vi "FPGA - Main.vi"() -> ()   [LabVIEW 2017]
uses:
  <vilib>/rvi/Emulation/niFpgaGetClockAttributes.vi
  <vilib>/rvi/Emulation/niFpgaSctlEmulationGetInTimedLoop.vi
  <vilib>/rvi/Emulation/niFpgaEmulationReportErrorSimple.vi
  <vilib>/rvi/eio/common/nirviEmuTemplateMethod_errors.vi
  <vilib>/rvi/interface/RandomDataEmulation/niFpgaRandomDataHandleErrors.vi
  <vilib>/rvi/Emulation/niFpgaCriticalErrorInLSC.vi
  <vilib>/eio/EIONode/EIONode.xnode
  <vilib>/rvi/DataTransferAndStorage/Container/XNode/niFpgaContainer.xnode
  <vilib>/rvi/interface/RandomDataEmulation/nirviRandomDataFpgaReadWriteTemplate.vi
panel:
  in  "Manual Log":bool
  in  "Reset":bool
  out "Loop Iteration":i32
  out "Delay":u32
  out "Data":u32[](array[numeric])
  in  "Wait(uSec)":u32
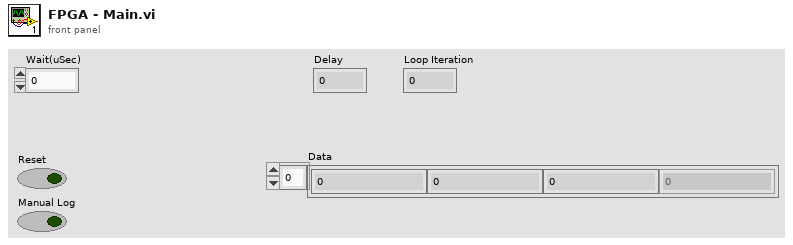
[diagram p1: front panel]
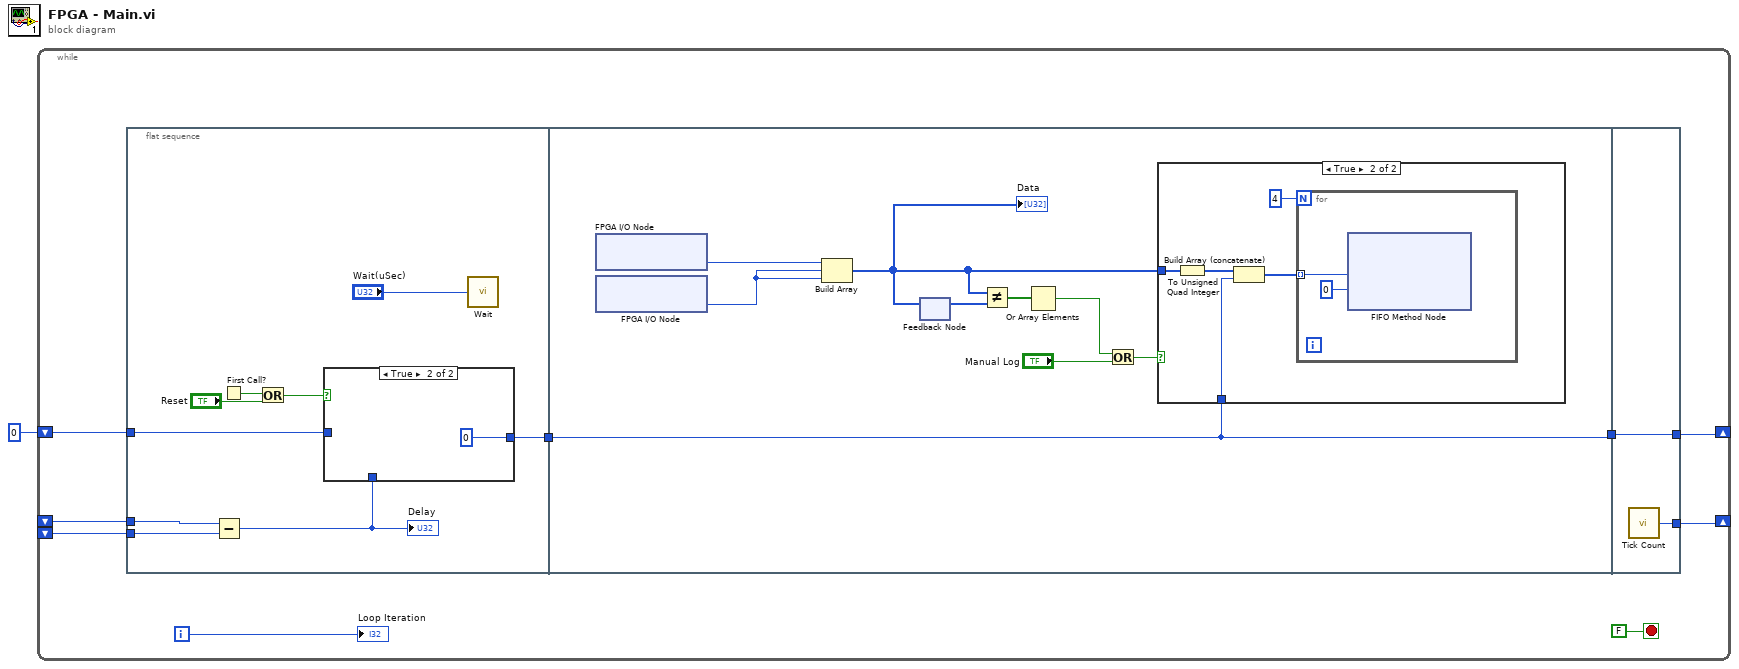
[diagram p0: block diagram]
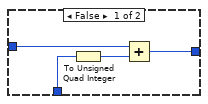
[diagram p2: hidden frame]
diagram:
  n1 = while {
    shift-right: [w9] -> _
    shift-left: _ -> [w8]
    shift-left: _ -> [w7]
    shift-right: [w2] -> _
    shift-left: u64 0 ("x-y") -> [w5]
    i -> [w6]
    stop <- FALSE stop-if-true
    n2 = flat-sequence {
      tunnel: w8 -> [w18]
      tunnel: w7 -> [w17]
      tunnel: w5 -> [w15]
      tunnel: [w14] -> w4
      tunnel: w4 -> [w29]
      tunnel: [w29] -> w3
      tunnel: [w42] -> w9
      tunnel: w3 -> [w41]
      tunnel: [w41] -> w2
      frame #0 {
        n3 = Subtract(x=w18, y=w17) -> (x-y=w16:u32)
        "Delay" <- w16
        n4 = First Call?() -> (First Call?: T/F=w13:bool)
        n5 = Or(x=w13, y="Reset") -> (x .or. y?=w11:bool)
        n6 = case shown="True" w11 {
          tunnel: w16 -> [w23 _]
          tunnel: w15 -> [w22 _]
          tunnel: [w21 u64 0] -> w14
          frame False {
            n7 = To Unsigned Quad Integer(1:w23) -> (0:w20:u64)
            n8 = Add(x=w22, y=w20) -> (x+y=w21:u64)
          }
          frame True {
          }
        }
        n9 = call "Wait"("Count(uSec)"="Wait(uSec)") -> ()  [unwired: 1 out]
      }
      frame #1 {
        n10 = xnode "FPGA I/O Node"() -> ("Mod1/DI31:0"=w33:u32)  [unwired: 1 in, 1 out]
        n11 = xnode "FPGA I/O Node"() -> ("Mod2/DI31:0"=w25:u32)  [unwired: 1 in, 1 out]
        n12 = Build Array(w33, w25, w25) -> (w31:u32[])
        "Data" <- w31
        n13 = feedback-in #1(w31) -> ()
        n14 = feedback #1() -> (w32:u32[])  [unwired: 1 in]
        n15 = Not Equal?(x=w31, y=w32) -> (x != y?=w30:bool[])
        n16 = Or Array Elements(Boolean array=w30) -> (logical OR=w28:bool)
        n17 = Or(x=w28, y="Manual Log") -> (x .or. y?=w26:bool)
        n18 = case shown="True" w26 {
          tunnel: w31 -> [_ w37]
          tunnel: w29 -> [_ w36]
          frame False {
          }
          frame True {
            n19 = To Unsigned Quad Integer(1:w37) -> (0:w34:u64[])
            n20 = Build Array (concatenate)(w34, w36) -> (w35:u64[])
            n21 = for {
              N: 4 -> [_]
              tunnel: w35 -> [w40] mode=indexing
              n22 = xnode ("FIFO Method Node")("Element"=w40, "Timeout"=0) -> ()  [unwired: 1 in, 2 out]
            }
          }
        }
      }
      frame #2 {
        n23 = call "Tick Count"() -> ("Tick Count(uSec)"=w42:u32)
      }
    }
    "Loop Iteration" <- w6
  }
